vi "Sup.vi"(9 "f":dbl, 11 "array":dbl[](array[numeric])=[0.0]) -> (1 "sup_index":i32, 3 "sup_value":dbl)   [LabVIEW 2014]
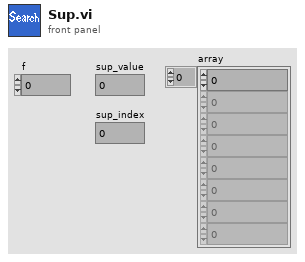
[diagram p1: front panel]
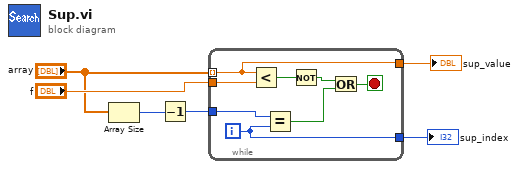
[diagram p0: block diagram]
diagram:
  n1 = Array Size(array="array") -> (size(s)=w5:i32)
  n2 = Decrement(x=w5) -> (x-1=w4:i32)
  n3 = while {
    tunnel: "array" -> [w7] mode=indexing
    tunnel: "f" -> [w14]
    tunnel: w4 -> [w13]
    tunnel: [w8] -> w2
    tunnel: [w7] -> w1
    i -> [w8]
    stop <- w11 stop-if-true
    n4 = Less?(x=w7, y=w14) -> (x < y?=w10:bool)
    n5 = Equal?(x=w13, y=w8) -> (x = y?=w12:bool)
    n6 = Not(x=w10) -> (.not. x?=w9:bool)
    n7 = Or(x=w9, y=w12) -> (x .or. y?=w11:bool)
  }
  "sup_index" <- w2
  "sup_value" <- w1
